vi "Dlg-Select Existing Version.vi"(8 "error in (no error)":errorcluster, 11 "Strings []":string[](array[string])) -> (0 "error in (no error) (dup)":errorcluster, 2 "selected version":string, 3 "cancelled?":bool)   [LabVIEW 2013]
panel:
  in  "Cancel":bool
  in  "OK":bool
  in  "LabVIEW List":string(combo)
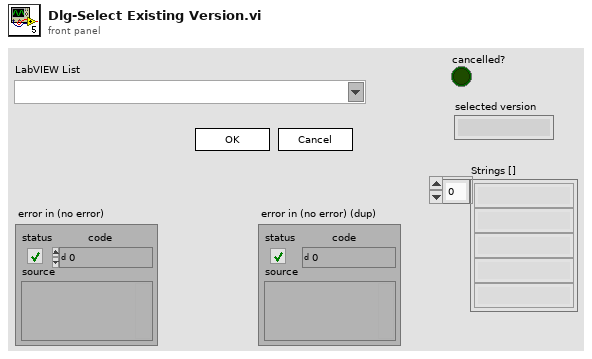
[diagram p1: front panel]
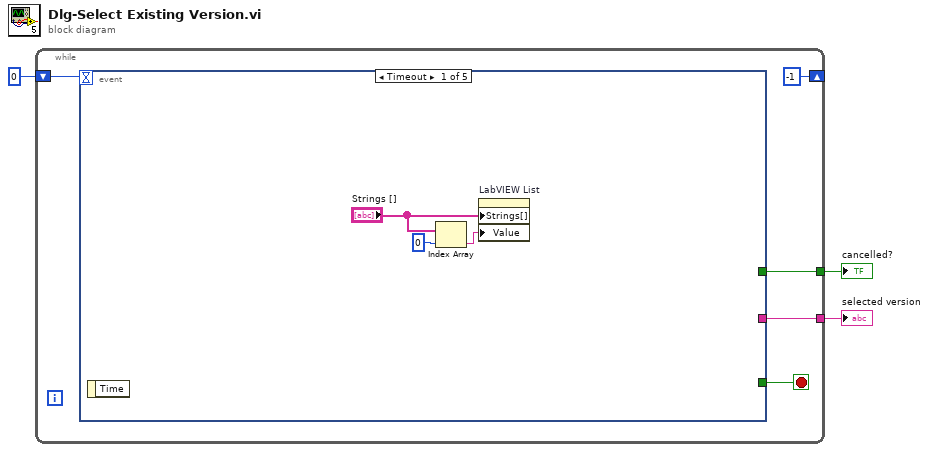
[diagram p0: block diagram]
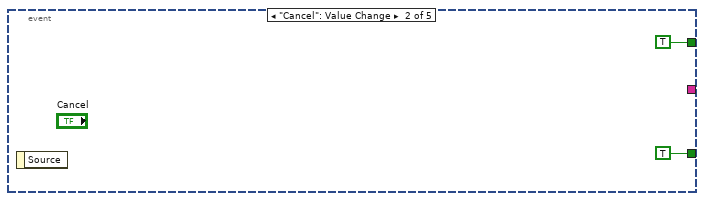
[diagram p2: hidden frame]
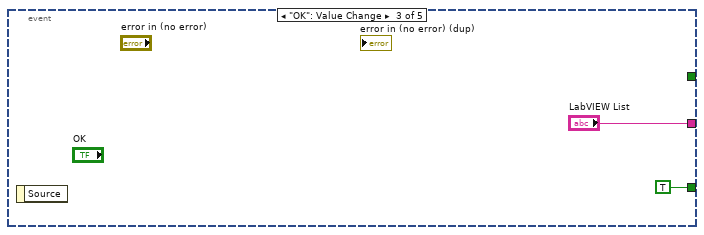
[diagram p3: hidden frame]
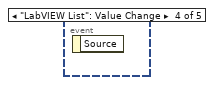
[diagram p4: hidden frame]
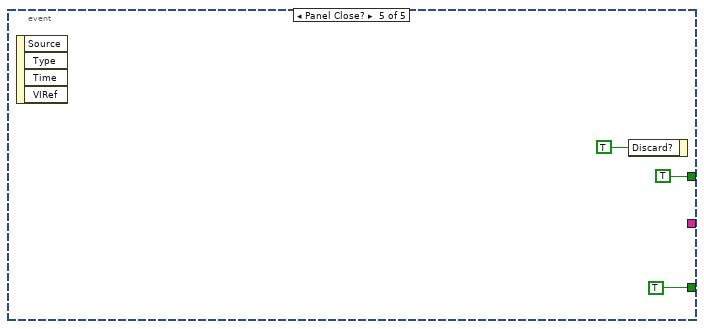
[diagram p5: hidden frame]
diagram:
  n1 = while {
    shift-right: [-1] -> _
    shift-left: 0 -> [w7]
    tunnel: [w5] -> w2
    tunnel: [w4] -> w1
    stop <- w8 stop-if-true
    n2 = event shown="[0] Timeout" {
      selector: _ -> [_ _ _ _ _]
      dyn-events: _ -> [_ _ _ _ _]
      timeout: w7 -> [_ _ _ _ _]
      tunnel: [_ TRUE ("Discard?") TRUE ("Discard?") _ TRUE ("Discard?")] -> w8
      tunnel: [_ _ "LabVIEW List" _ _] -> w5
      tunnel: [_ TRUE ("Discard?") _ _ TRUE ("Discard?")] -> w4
      event Timeout {
        n3 = event-data() -> ()  [unwired: 1 in, 1 out]
        n4 = Index Array(array="Strings []", index=0) -> (element=w11:string)
        n5 = property on="LabVIEW List" class="CmbBox"("Strings[]"="Strings []", "Value"=w11) -> ()  [unwired: 2 in, 2 out]
      }
      event "Cancel": Value Change {
        n6 = event-data() -> ()  [unwired: 1 in, 1 out]
      }
      event "OK": Value Change {
        n7 = event-data() -> ()  [unwired: 1 in, 1 out]
      }
      event "LabVIEW List": Value Change {
        n8 = event-data() -> ()  [unwired: 1 in, 1 out]
      }
      event Panel Close? {
        n9 = event-data() -> ()  [unwired: 1 in, 4 out]
        n10 = event-data("Discard?"=TRUE) -> ()  [unwired: 1 in, 1 out]
      }
    }
  }
  "selected version" <- w2
  "cancelled?" <- w1
